vi "Check Analog Data Sync.vi"(8 "error in (no error)":errorcluster, 10 "Analog Data":sgl[][](array[numeric])) -> (0 "error out":errorcluster, 2 "Analog Data Out":sgl[][](array[numeric]))   [LabVIEW 2020]
uses:
  Type Definitions/Enum - Notification Types.ctl
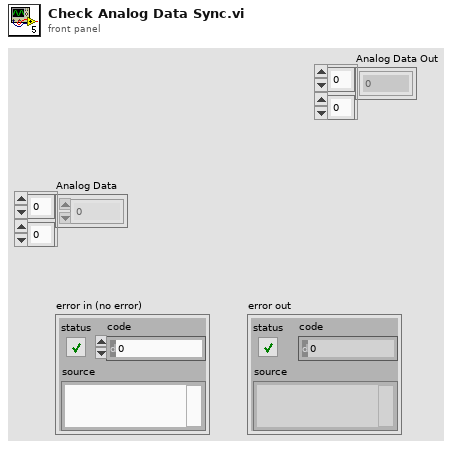
[diagram p1: front panel]
types:
  T1 = typedef "Enum - Notification Types.ctl" = enum16{"Warning", "Acknowledge", "Notification"}
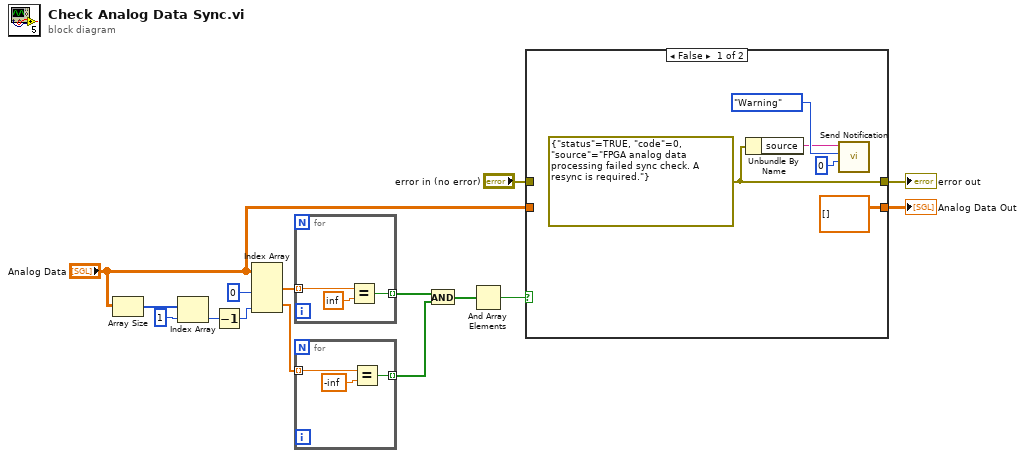
[diagram p0: block diagram]
diagram:
  n1 = Array Size(array="Analog Data") -> (size(s)=w4:i32[])
  n2 = Index Array(array=w4, index=1) -> (element=w8:i32)
  n3 = Decrement(x=w8) -> (x-1=w5:i32)
  n4 = Index Array(array="Analog Data", index (col) #1=0 ("disabled index (col)"), index (col) #2=w5) -> (element #1=w6:sgl[], element #2=w9:sgl[])  [unwired: 2 in]
  n5 = for {
    tunnel: w6 -> [w18] mode=indexing
    tunnel: [w16] -> w10 mode=indexing
    n6 = Equal?(x=w18, y=sgl inf) -> (x = y?=w16:bool)
  }
  n7 = for {
    tunnel: w9 -> [w21] mode=indexing
    tunnel: [w19] -> w11 mode=indexing
    n8 = Equal?(x=w21, y=sgl -inf) -> (x = y?=w19:bool)
  }
  n9 = And(x=w10, y=w11) -> (x .and. y?=w12:bool[])
  n10 = And Array Elements(Boolean array=w12) -> (logical AND=w13:bool)
  n11 = case shown="False" w13 {
    tunnel: "error in (no error)" -> [_ w28]
    tunnel: [w23 w28] -> w15
    tunnel: "Analog Data" -> [_ w27]
    tunnel: [sgl[][] [] ("Analog Data") w27] -> w1
    frame False {
      w23 = errorcluster {"status"=TRUE, "code"=0, "source"="FPGA analog data processing failed sync check. A resync is required."} ("error out")
      n12 = Unbundle By Name(w23) -> ("source"=w22:string)
      n13 = call "Send Notification.vi"("Code (0)"=0, "Notification Type (Notification)"=Enum_-_Notification_Types."Warning", "Description (\"\")"=w22) -> ()  [unwired: 7 in, 2 out]
    }
    frame True {
      # "Pass Sync Check"
    }
  }
  "error out" <- w15
  "Analog Data Out" <- w1
